vi "74hc194.vi"(0 "cp":bool, 1 "CR`":bool, 2 "S0":bool, 3 "S1":bool, 4 "Dsr":bool, 5 "Dsl":bool, 6 "D1":bool, 7 "D2":bool, 8 "D0":bool, 9 "D3":bool) -> (15 "Q0":bool, 16 "Q1":bool, 17 "Q2":bool, 18 "Q3":bool)   [LabVIEW 2018]
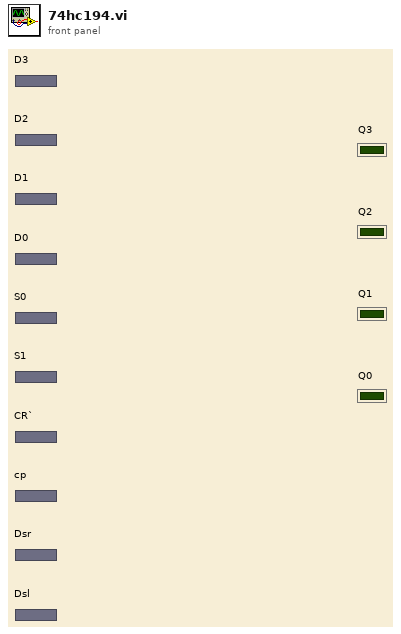
[diagram p1: front panel]
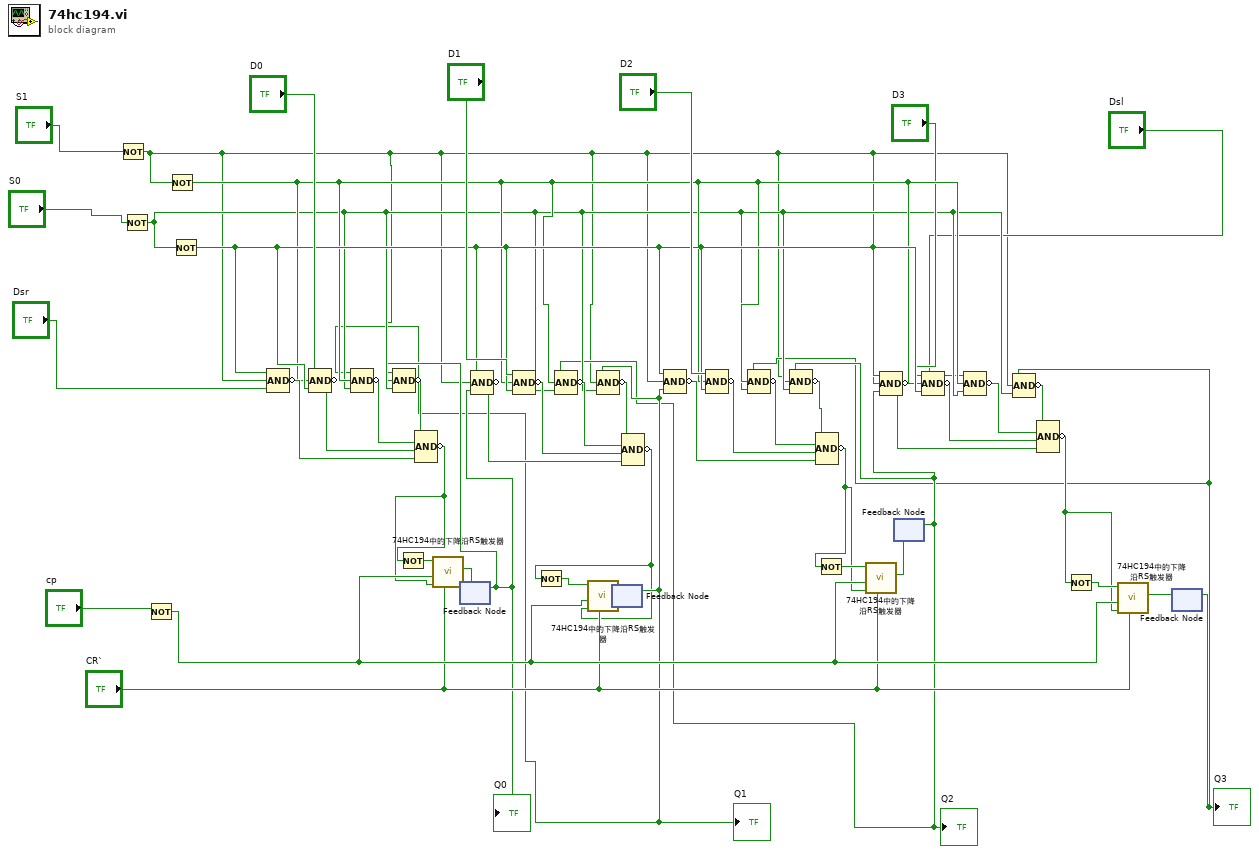
[diagram p0: block diagram]
diagram:
  n1 = Not(x="S1") -> (.not. x?=w1:bool)
  n2 = Not(x="S0") -> (.not. x?=w22:bool)
  n3 = Not(x="cp") -> (.not. x?=w15:bool)
  n4 = Not(x=w1) -> (.not. x?=w24:bool)
  n5 = Not(x=w22) -> (.not. x?=w25:bool)
  n6 = Compound Arithmetic op=AND ("复合运算")(w25, w1, "Dsr") -> (invert w45:bool)
  n7 = Compound Arithmetic op=AND ("复合运算")("D0", w24, w25) -> (invert w44:bool)
  n8 = feedback #1() -> (w12:bool)  [unwired: 1 in]
  "Q0" <- w12
  n9 = Compound Arithmetic op=AND ("复合运算")(w12, w1, w22) -> (invert w42:bool)
  n10 = Compound Arithmetic op=AND ("复合运算")(w25, w1, w12) -> (invert w41:bool)
  n11 = Compound Arithmetic op=AND ("复合运算")("D1", w24, w25) -> (invert w40:bool)
  n12 = feedback #2() -> (w10:bool)  [unwired: 1 in]
  "Q1" <- w10
  n13 = Compound Arithmetic op=AND ("复合运算")(w10, w24, w22) -> (invert w43:bool)
  n14 = Compound Arithmetic op=AND ("复合运算")(w42, w43, w44, w45) -> (invert w9:bool)
  n15 = Not(x=w9) -> (.not. x?=w20:bool)
  n16 = call "74HC194中的下降沿RS触发器.vi"("R0"="CR`", "R"=w9, "CP"=w15, "S"=w20) -> ("Q"=w13:bool)  [unwired: 7 in]
  n17 = feedback-in #1(w13) -> ()
  n18 = Compound Arithmetic op=AND ("复合运算")(w10, w1, w22) -> (invert w38:bool)
  n19 = Compound Arithmetic op=AND ("复合运算")(w25, w1, w10) -> (invert w37:bool)
  n20 = Compound Arithmetic op=AND ("复合运算")("D2", w24, w25) -> (invert w36:bool)
  n21 = feedback #3() -> (w4:bool)  [unwired: 1 in]
  "Q2" <- w4
  n22 = Compound Arithmetic op=AND ("复合运算")(w4, w24, w22) -> (invert w39:bool)
  n23 = Compound Arithmetic op=AND ("复合运算")(w38, w39, w40, w41) -> (invert w8:bool)
  n24 = Not(x=w8) -> (.not. x?=w19:bool)
  n25 = call "74HC194中的下降沿RS触发器.vi"("R0"="CR`", "R"=w8, "CP"=w15, "S"=w19) -> ("Q"=w11:bool)  [unwired: 7 in]
  n26 = feedback-in #2(w11) -> ()
  n27 = Compound Arithmetic op=AND ("复合运算")(w4, w1, w22) -> (invert w34:bool)
  n28 = Compound Arithmetic op=AND ("复合运算")(w25, w1, w4) -> (invert w33:bool)
  n29 = Compound Arithmetic op=AND ("复合运算")("D3", w24, w25) -> (invert w32:bool)
  n30 = Compound Arithmetic op=AND ("复合运算")("Dsl", w24, w22) -> (invert w31:bool)
  n31 = feedback #4() -> (w2:bool)  [unwired: 1 in]
  "Q3" <- w2
  n32 = Compound Arithmetic op=AND ("复合运算")(w2, w24, w22) -> (invert w35:bool)
  n33 = Compound Arithmetic op=AND ("复合运算")(w34, w35, w36, w37) -> (invert w7:bool)
  n34 = Not(x=w7) -> (.not. x?=w17:bool)
  n35 = call "74HC194中的下降沿RS触发器.vi"("R0"="CR`", "R"=w7, "CP"=w15, "S"=w17) -> ("Q"=w5:bool)  [unwired: 7 in]
  n36 = feedback-in #3(w5) -> ()
  n37 = Compound Arithmetic op=AND ("复合运算")(w2, w1, w22) -> (invert w30:bool)
  n38 = Compound Arithmetic op=AND ("复合运算")(w30, w31, w32, w33) -> (invert w6:bool)
  n39 = Not(x=w6) -> (.not. x?=w18:bool)
  n40 = call "74HC194中的下降沿RS触发器.vi"("R0"="CR`", "R"=w6, "CP"=w15, "S"=w18) -> ("Q"=w3:bool)  [unwired: 7 in]
  n41 = feedback-in #4(w3) -> ()
